vi "TD.vi"(8 "error in (no error)":errorcluster, 10 "Sine":waveform(dbl)[](graph)) -> (0 "error out":errorcluster, 2 "TD (%)":dbl=5.0)   [LabVIEW 2019, in "Prueba21.lvclass"]
uses:
  Prueba21.lvclass
  <vilib>/measure/matone.llb/Harmonic Distortion Analyzer N Chan.vi
  <vilib>/measure/NI_MAPro.lvlib
panel:
  out "THD (%)":dbl[](array[numeric])
  out "Armonicos":dbl[](array[numeric])
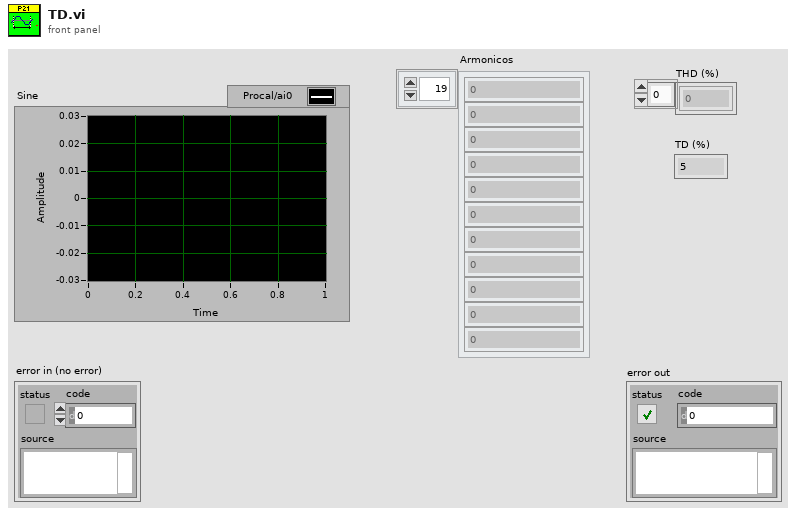
[diagram p1: front panel]
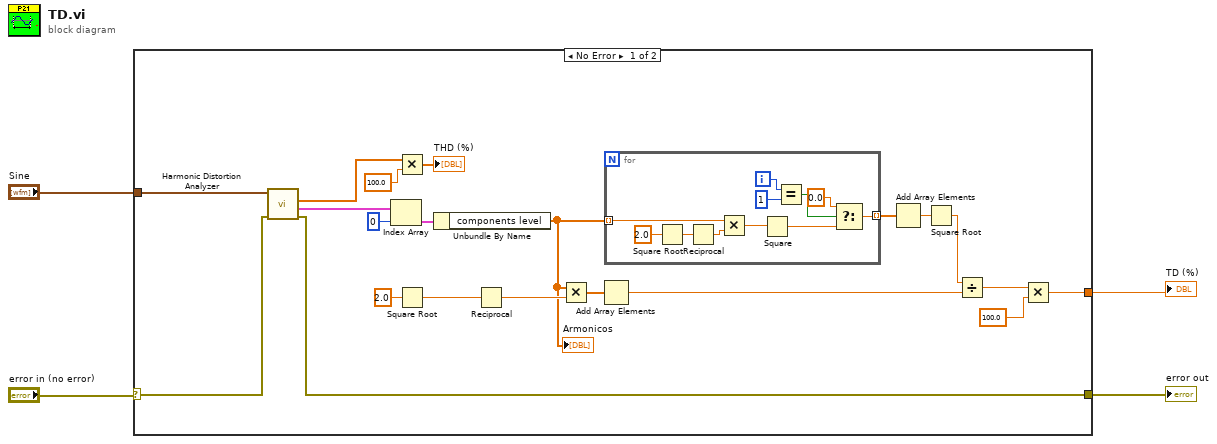
[diagram p0: block diagram]
diagram:
  n1 = case shown="No Error" "error in (no error)" {
    selector: "error in (no error)" -> [w5 w37]
    tunnel: [w6 w37] -> w3
    tunnel: "Sine" -> [w8 _]
    tunnel: [w7 _] -> w1
    frame No Error {
      n2 = call-poly <vilib>:"Harmonic Distortion Analyzer.vi"("error in (no error)"=w5, "signals in"=w8) -> ("error out"=w6:errorcluster, "components levels"=w13:cluster{"components level":dbl[]}[], "THD"=w25:dbl[])  [unwired: 4 in, 3 out]
      n3 = Index Array(array=w13, index=0) -> (element=w11:cluster{"components level":dbl[]})
      n4 = Multiply(x=w25, y=100.0) -> (x*y=→"THD (%)":dbl[])
      n5 = Square Root(x=2.0) -> (sqrt(x)=w20:dbl)
      n6 = Unbundle By Name(w11) -> ("components level"=w10:dbl[])
      "Armonicos" <- w10
      n7 = Reciprocal(x=w20) -> (1/x=w17:dbl)
      n8 = Multiply(x=w10, y=w17) -> (x*y=w18:dbl[])
      n9 = Add Array Elements(numeric array=w18) -> (sum=w23:dbl)
      n10 = for {
        tunnel: w10 -> [w29] mode=indexing
        tunnel: [w32] -> w16 mode=indexing
        i -> [w36]
        n11 = Square Root(x=2.0) -> (sqrt(x)=w30:dbl)
        n12 = Reciprocal(x=w30) -> (1/x=w28:dbl)
        n13 = Multiply(x=w29, y=w28) -> (x*y=w27:dbl)
        n14 = Square(x=w27) -> (x^2=w26:dbl)
        n15 = Equal?(x=w36, y=1) -> (x = y?=w34:bool)
        n16 = Select(t=0.0, s=w34, f=w26) -> (s? t:f=w32:dbl)
      }
      n17 = Add Array Elements(numeric array=w16) -> (sum=w15:dbl)
      n18 = Square Root(x=w15) -> (sqrt(x)=w14:dbl)
      n19 = Divide(x=w14, y=w23) -> (x/y=w22:dbl)
      n20 = Multiply(x=w22, y=100.0) -> (x*y=w7:dbl)
    }
    frame Error {
    }
  }
  "error out" <- w3
  "TD (%)" <- w1
